vi "CFD_reduced.vi"(8 "Delay Array":dbl[](array[numeric]), 10 "Attenuation":dbl, 11 "Waveform_in":waveform(dbl)) -> (0 "not_detected":bool, 3 "CFD":i32)   [LabVIEW 2019]
uses:
  <vilib>/Analysis/3filter.llb/Savitzky-Golay Filter (DBL).vi
  SiPM_Tests_Global_Var.vi
  <vilib>/Analysis/NI_AALBase.lvlib
  <vilib>/ptbypt/NI_PtbyPt.lvlib
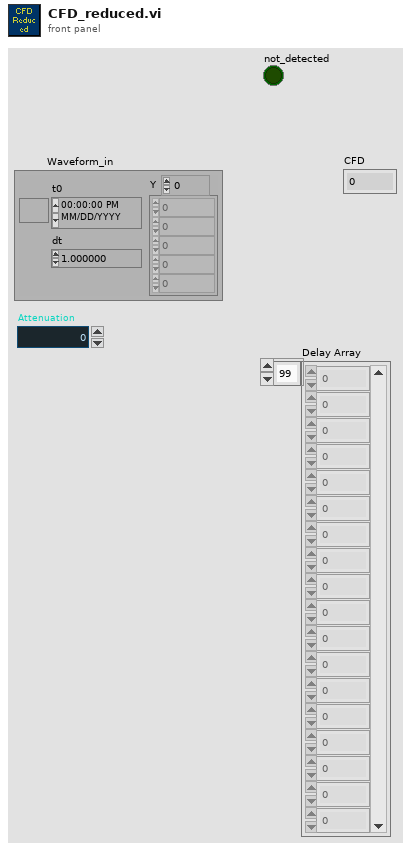
[diagram p1: front panel]
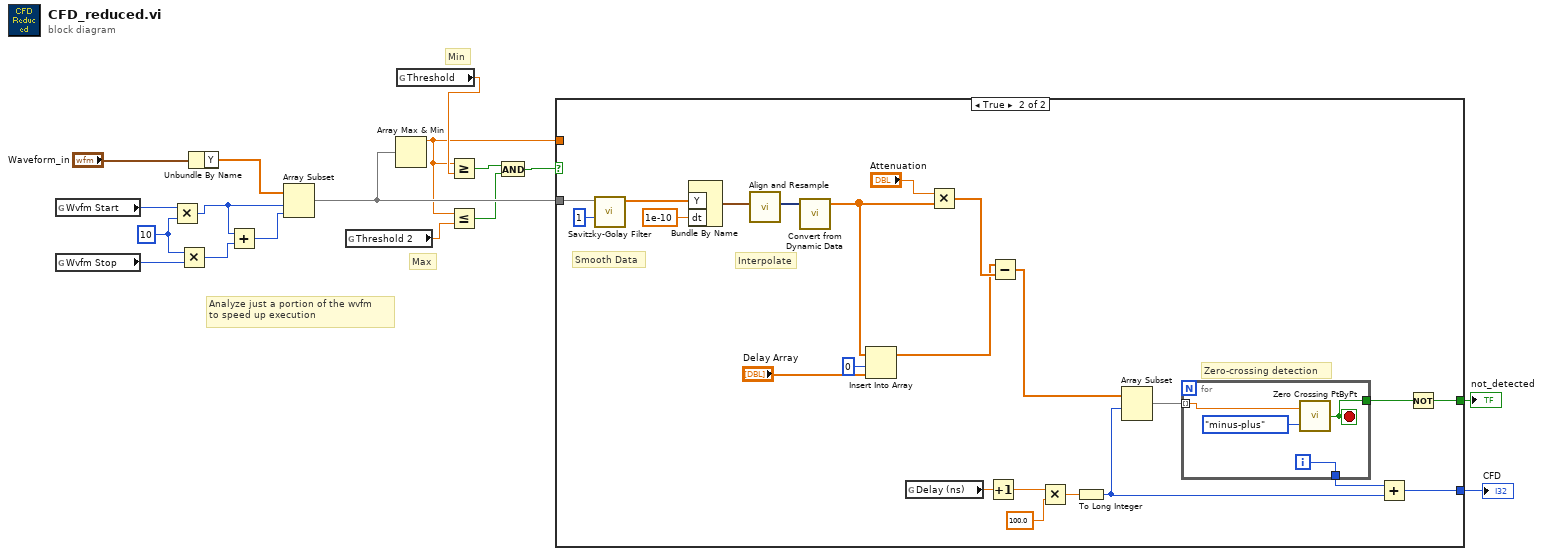
[diagram p0: block diagram]
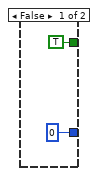
[diagram p2: hidden frame]
diagram:
  w16 = 10 ("y")
  # "Max"
  # "Min"
  # "Analyze just a portion of the wvfm \nto speed up execution"
  n1 = global read "SiPM_Tests_Global_Var.vi" "Wvfm Start"() -> (w17:i32)
  n2 = global read "SiPM_Tests_Global_Var.vi" "Wvfm Stop"() -> (w15:i32)
  n3 = Multiply(x=w17, y=w16) -> (x*y=w14:i32)
  n4 = Multiply(x=w16, y=w15) -> (x*y=w13:i32)
  n5 = Unbundle By Name("Waveform_in") -> ("Y"=w9:dbl[])
  n6 = Add(x=w14, y=w13) -> (x+y=w12:i32)
  n7 = Array Subset(array=w9, index=w14, length=w12) -> (w11:dbl[])
  n8 = global read "SiPM_Tests_Global_Var.vi" "Threshold 2"() -> (w7:dbl)
  n9 = Array Max & Min(array=w11) -> (max value=w8:dbl)  [unwired: 3 out]
  n10 = global read "SiPM_Tests_Global_Var.vi" "Threshold"() -> (w10:dbl)
  n11 = Greater Or Equal?(x=w8, y=w10) -> (x >= y?=w6:bool)
  n12 = Less Or Equal?(x=w8, y=w7) -> (x <= y?=w4:bool)
  n13 = And(x=w6, y=w4) -> (x .and. y?=w5:bool)
  n14 = case shown="True" w5 {
    tunnel: w11 -> [_ w34]
    tunnel: [0 w25] -> w2
    tunnel: w8 -> [_ _]
    tunnel: [TRUE w20] -> w1
    frame False {
    }
    frame True {
      # "Zero-crossing detection"
      # "Interpolate"
      # "Smooth Data"
      n15 = call-poly <vilib>:"Savitzky-Golay Filter.vi"("polynomial order"=1, "X"=w34) -> ("Filtered X"=w37:dbl[])  [unwired: 8 in, 1 out]
      n16 = Bundle By Name("Y"=w37, "dt"=1e-10) -> (w38:waveform(dbl))  [unwired: 1 in]
      n17 = call "Align and Resample"("Signals"=w38) -> ("Resampled Signals"=w41:dynamicdata)  [unwired: 8 in, 2 out]
      n18 = call "Convert from Dynamic Data"("Dynamic Data Type"=w41) -> ("Array"=w24:dbl[])  [unwired: 3 in]
      n19 = Insert Into Array(array=w24, index=0, new element="Delay Array") -> (w35:dbl[])
      n20 = global read "SiPM_Tests_Global_Var.vi" "Delay (ns)"() -> (w31:dbl)
      n21 = Multiply(x="Attenuation", y=w24) -> (x*y=w36:dbl[])
      n22 = Increment(x=w31) -> (x+1=w30:dbl)
      n23 = Subtract(x=w35, y=w36) -> (x-y=w33:dbl[])
      n24 = Multiply(x=w30, y=100.0) -> (x*y=w29:dbl)
      n25 = To Long Integer(number=w29) -> (32bit integer=w28:i32)
      n26 = Array Subset(array=w33, index=w28) -> (w27:dbl[])  [unwired: 1 in]
      n27 = for {
        tunnel: w27 -> [w45] mode=indexing
        tunnel: [w44] -> w26
        tunnel: [w43] -> w21
        i -> [w44]
        stop <- w43 stop-if-true
        n28 = call <vilib>:"Zero Crossing PtByPt.vi"("direction"=enum16{"either", "minus-plus", "plus-minus"}."minus-plus", "input data point"=w45) -> ("crossing"=w43:bool)  [unwired: 1 in]
      }
      n29 = Add(x=w26, y=w28) -> (x+y=w25:i32)
      n30 = Not(x=w21) -> (.not. x?=w20:bool)
    }
  }
  "CFD" <- w2
  "not_detected" <- w1
